vi "meth.OutputLoop.vi"(0 "class.GLue in":refnum<class "class.GLue.lvclass">, 7 "ReaderContext in":T1, 11 "error in":errorcluster) -> (4 "class.GLue out":refnum<class "class.GLue.lvclass">, 15 "error out":errorcluster)   [LabVIEW 2014, in "GLue.lvlib" / "class.GLue.lvclass"]
uses:
  class.GLue.lvclass
  class.GLue.lvclass/class.GLue.ctl
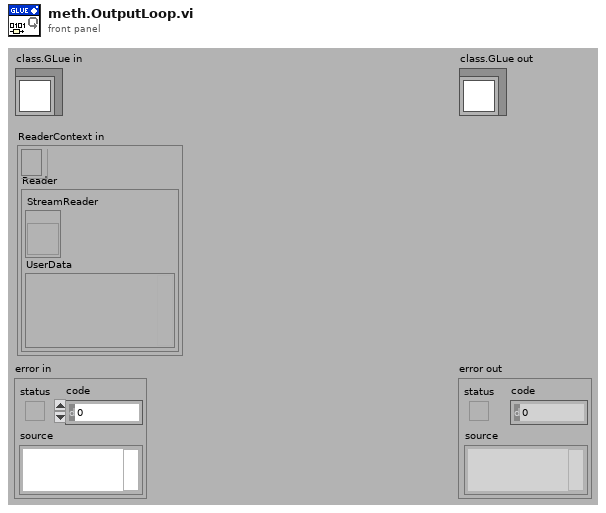
[diagram p1: front panel]
types:
  T1 = cluster{"EventRef":refnum<event-registration>, "Reader":cluster{"StreamReader":refnum<vi>, "UserData":variant}}
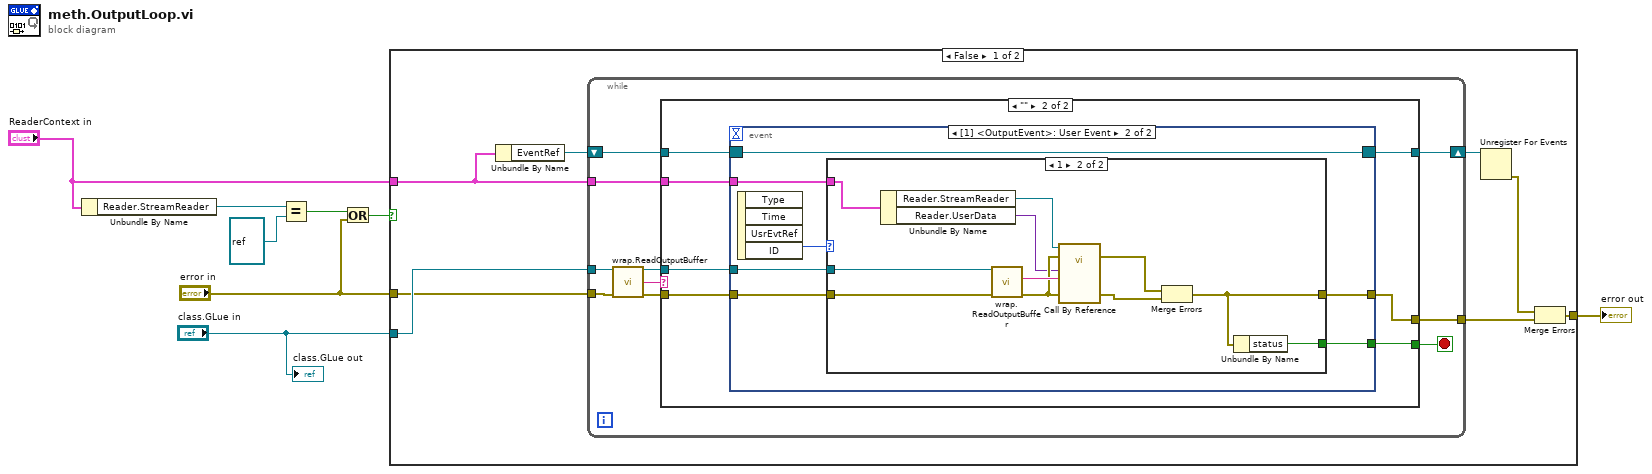
[diagram p0: block diagram]
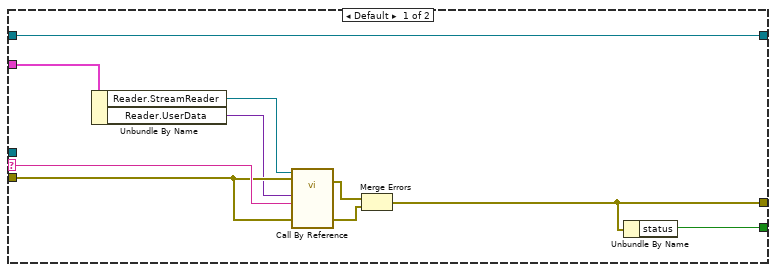
[diagram p2: hidden frame]
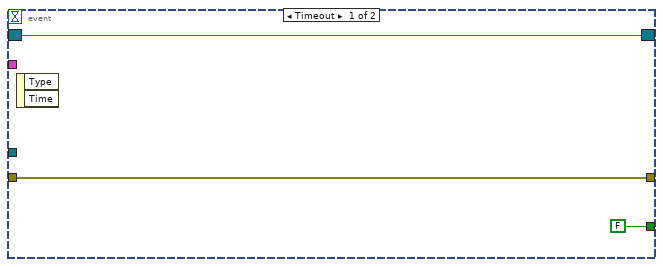
[diagram p3: hidden frame]
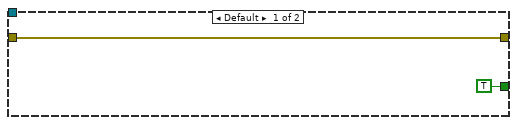
[diagram p4: hidden frame]
diagram:
  n1 = Unbundle By Name("ReaderContext in") -> ("Reader.StreamReader"=w3:refnum<vi>)
  n2 = Equal?(x=w3, y=refnum<vi> refnum ("Reader.StreamReader")) -> (x = y?=w7:bool)
  n3 = Or(x=w7, y="error in") -> (x .or. y?=w6:bool)
  n4 = case shown="False" w6 {
    tunnel: "class.GLue in" -> [w16 _]
    tunnel: "error in" -> [w11 w67]
    tunnel: [w12 w67] -> w5
    tunnel: "ReaderContext in" -> [w9 _]
    frame False {
      n5 = Unbundle By Name(w9) -> ("EventRef"=w10:refnum<event-registration>)
      n6 = while {
        tunnel: w11 -> [w26]
        tunnel: w16 -> [w25]
        tunnel: [w22] -> w13
        tunnel: w9 -> [w17]
        shift-right: [w18] -> w15
        shift-left: w10 -> [w19]
        stop <- w21 stop-if-true
        n7 = call "wrap.ReadOutputBuffer.vi"("class.GLue in"=w25, "error in (no error)"=w26) -> ("class.GLue out"=w20:refnum<class "class.GLue.lvclass">, "String"=w24:string, "error out"=w23:errorcluster)  [unwired: 11 in]
        n8 = case shown="\"\"" w24 {
          selector: w24 -> [w36 _]
          tunnel: w23 -> [w35 w40]
          tunnel: [w32 w39] -> w22
          tunnel: [w31 w38] -> w21
          tunnel: w20 -> [_ w41]
          tunnel: w19 -> [w30 w43]
          tunnel: [w30 w42] -> w18
          tunnel: w17 -> [w29 w37]
          frame Default {
            n9 = Unbundle By Name(w29) -> ("Reader.StreamReader"=w28:refnum<vi>, "Reader.UserData"=w27:variant)
            n10 = call-by-ref "?"(reference=w28, error in=w35, 8:"error in (no error)"=w35, "String"=w36, "variant"=w27) -> (error out=w34:errorcluster, 0:"error out"=w33:errorcluster)  [unwired: 8 in, 1 out]
            n11 = Merge Errors(w34, w33) -> (w32:errorcluster)
            n12 = Unbundle By Name(w32) -> ("status"=w31:bool)
          }
          frame "" {
            n13 = event shown="[1] <OutputEvent>: User Event" {
              selector: w43 -> [w46 w53]
              dyn-events: [w46 w53] -> w42
              timeout: _ -> [_ _]
              tunnel: w41 -> [_ w51]
              tunnel: w40 -> [w45 w50]
              tunnel: [w45 w49] -> w39
              tunnel: [FALSE w48] -> w38
              tunnel: w37 -> [_ w47]
              event Timeout {
                n14 = event-data() -> ()  [unwired: 1 in, 2 out]
              }
              event User Event {
                n15 = event-data() -> ("ID"=w52:i32)  [unwired: 1 in, 3 out]
                n16 = case shown="1" w52 {
                  tunnel: w51 -> [_ w66]
                  tunnel: w50 -> [w55 w65]
                  tunnel: [w55 w60] -> w49
                  tunnel: [TRUE ("status") w59] -> w48
                  tunnel: w47 -> [_ w58]
                  frame Default {
                  }
                  frame 1 {
                    n17 = Unbundle By Name(w58) -> ("Reader.StreamReader"=w57:refnum<vi>, "Reader.UserData"=w56:variant)
                    n18 = call "wrap.ReadOutputBuffer.vi"("class.GLue in"=w66, "error in (no error)"=w65) -> ("String"=w62:string, "error out"=w61:errorcluster)  [unwired: 11 in, 1 out]
                    n19 = call-by-ref "?"(reference=w57, error in=w61, 8:"error in (no error)"=w61, "String"=w62, "variant"=w56) -> (error out=w64:errorcluster, 0:"error out"=w63:errorcluster)  [unwired: 8 in, 1 out]
                    n20 = Merge Errors(w64, w63) -> (w60:errorcluster)
                    n21 = Unbundle By Name(w60) -> ("status"=w59:bool)
                  }
                }
              }
            }
          }
        }
      }
      n22 = Unregister For Events(event registration refnum=w15) -> (error out=w14:errorcluster)  [unwired: 1 in]
      n23 = Merge Errors(w14, w13) -> (w12:errorcluster)
    }
    frame True {
    }
  }
  "error out" <- w5
  "class.GLue out" <- "class.GLue in"
